vi "Remove Between Cursors.vi"(6 "Left":dbl, 7 "Right":dbl, 8 "error in (no error)":errorcluster, 9 "Flow":dynamicdata(waveform), 10 "Pressure":dynamicdata(waveform), 11 "Audio":dynamicdata(waveform)) -> (0 "error out":errorcluster, 1 "Flow Clipped":dynamicdata(waveform), 2 "Pressure Clipped":dynamicdata(waveform), 3 "Audio Clipped":dynamicdata(waveform))   [LabVIEW 2020, in "AnalysisSupport.lvlib"]
uses:
  AnalysisSupport.lvlib
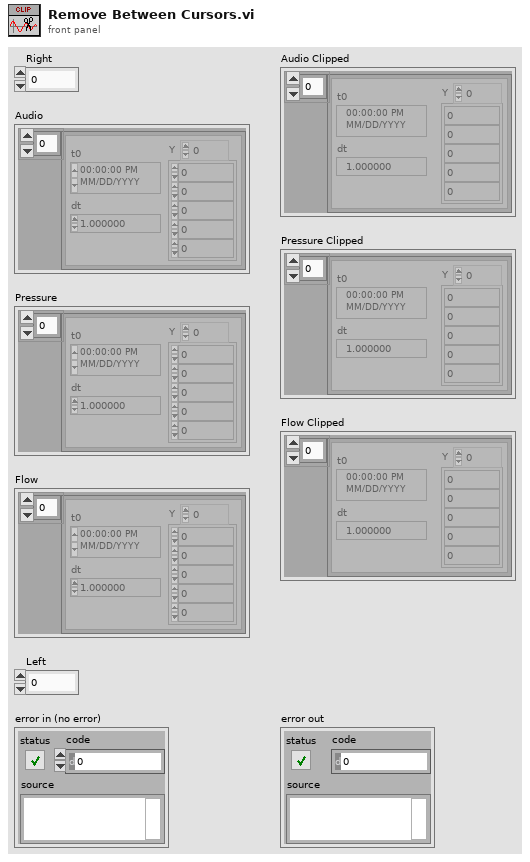
[diagram p1: front panel]
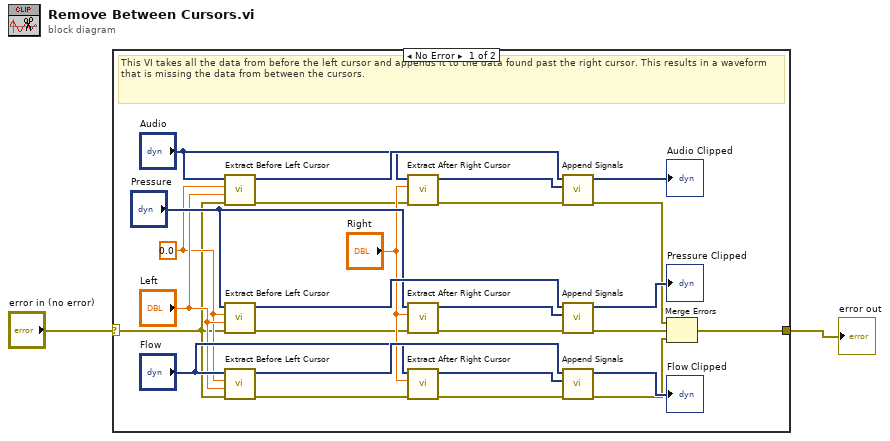
[diagram p0: block diagram]
diagram:
  n1 = case shown="No Error" "error in (no error)" {
    selector: "error in (no error)" -> [w3 w29]
    tunnel: [w4 w29] -> w2
    frame No Error {
      w14 = 0.0 ("Begin Offset")
      # "This VI takes all the data from before the left cursor and appends it to the data found past the right cursor. This results in a waveform that is missing the data from between the cursors."
      n2 = call "Extract Before Left Cursor"("error in (no error)"=w3, "Length"="Left", "Begin Offset"=w14, "Signals"="Audio") -> ("error out"=w5:errorcluster, "Section"=w8:dynamicdata)  [unwired: 6 in]
      n3 = call "Extract Before Left Cursor"("error in (no error)"=w3, "Length"="Left", "Begin Offset"=w14, "Signals"="Pressure") -> ("error out"=w15:errorcluster, "Section"=w23:dynamicdata)  [unwired: 6 in]
      n4 = call "Extract Before Left Cursor"("error in (no error)"=w3, "Length"="Left", "Begin Offset"=w14, "Signals"="Flow") -> ("error out"=w16:errorcluster, "Section"=w28:dynamicdata)  [unwired: 6 in]
      n5 = call "Extract After Right Cursor"("error in (no error)"=w5, "Begin Offset"="Right", "Signals"="Audio") -> ("error out"=w6:errorcluster, "Section"=w9:dynamicdata)  [unwired: 7 in]
      n6 = call "Extract After Right Cursor"("error in (no error)"=w15, "Begin Offset"="Right", "Signals"="Pressure") -> ("error out"=w18:errorcluster, "Section"=w24:dynamicdata)  [unwired: 7 in]
      n7 = call "Extract After Right Cursor"("error in (no error)"=w16, "Begin Offset"="Right", "Signals"="Flow") -> ("error out"=w17:errorcluster, "Section"=w27:dynamicdata)  [unwired: 7 in]
      n8 = call "Append Signals"("error in (no error)"=w6, "Input Signal B"=w9, "Input Signal A"=w8) -> ("error out"=w11:errorcluster, "Appended Signals"=→"Audio Clipped":dynamicdata)  [unwired: 7 in]
      n9 = call "Append Signals"("error in (no error)"=w18, "Input Signal B"=w24, "Input Signal A"=w23) -> ("error out"=w12:errorcluster, "Appended Signals"=→"Pressure Clipped":dynamicdata)  [unwired: 7 in]
      n10 = call "Append Signals"("error in (no error)"=w17, "Input Signal B"=w27, "Input Signal A"=w28) -> ("error out"=w13:errorcluster, "Appended Signals"=→"Flow Clipped":dynamicdata)  [unwired: 7 in]
      n11 = Merge Errors(w11, w12, w13) -> (w4:errorcluster)
    }
    frame Error {
    }
  }
  "error out" <- w2
